vi "Initialize.vi"(5 "instance":u8) -> (4 "subsystem":refnum<class "Single Address Space Collection.lvclass">, 6 "AddressSpace":refnum<class "AddressSpace.lvclass">)   [LabVIEW 2015, in "QuadEnc.lvlib" / "AddressSpace.lvclass"]
uses:
  AddressSpace.lvclass
  <instrlib>/_niInstr/Instruction Framework/v1/FPGA/Helper Classes/Single Address Space Collection/Single Address Space Collection.lvclass
  AddressSpace.lvclass/AddressSpace.ctl
  <vilib>/rvi/DataTransferAndStorage/Container/Common/niFpgaContainerGetUniqueNameForEmu.vi
  <vilib>/rvi/DataTransferAndStorage/Container/Common/niFpgaContainerSetEmuInfo.vi
  <vilib>/rvi/eio/common/nirviEmuReportErrorAndStop.vi
  <vilib>/rvi/LocalResourceManager/LocalResourceManager.xnode
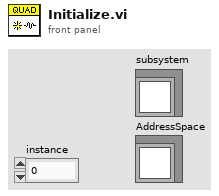
[diagram p1: front panel]
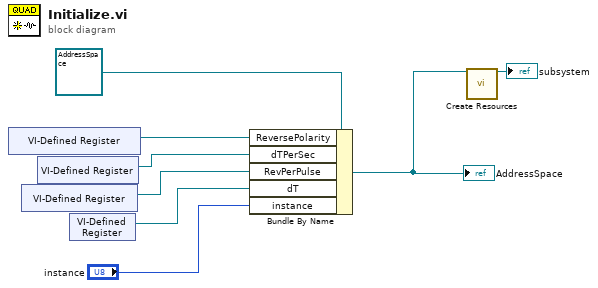
[diagram p0: block diagram]
diagram:
  n1 = xnode "VI-Defined Register"() -> ("Register Out"=w7:refnum<k21>)
  n2 = xnode "VI-Defined Register"() -> ("Register Out"=w5:refnum<k21>)
  n3 = xnode "VI-Defined Register"() -> ("Register Out"=w6:refnum<k21>)
  n4 = xnode "VI-Defined Register"() -> ("Register Out"=w4:refnum<k21>)
  n5 = Bundle By Name(cluster=refnum<class "AddressSpace.lvclass"> refnum ("QuadEnc.lvlib:AddressSpace.lvclass"), "ReversePolarity"=w7, "dTPerSec"=w6, "RevPerPulse"=w5, "dT"=w4, "instance"="instance") -> (w2:refnum<class "AddressSpace.lvclass">)
  "AddressSpace" <- w2
  n6 = call <instrlib>:"Create Resources.vi"("address space"=w2) -> ("single address space collection"=→"subsystem":refnum<class "Single Address Space Collection.lvclass">)  [unwired: 14 in]
